vi "Read Acceleration.vi"(8 "error in (no error)":errorcluster, 11 "Sync 2-Axis Stage Controller in":refnum<class "Sync 2-Axis Stage Controller.lvclass">) -> (0 "error out":errorcluster, 1 "Y Acceleration":dbl, 2 "X Acceleration":dbl, 3 "Sync 2-Axis Stage Controller out":refnum<class "Sync 2-Axis Stage Controller.lvclass">)   [LabVIEW 2022 SP3, in "Sync 2-Axis Stage Controller.lvclass"]
uses:
  Sync 2-Axis Stage Controller.lvclass
  Sync 2-Axis Stage Controller.lvclass/Sync 2-Axis Stage Controller.ctl
  Axis Objects/iMotion Controller/iMotion Controller.lvclass
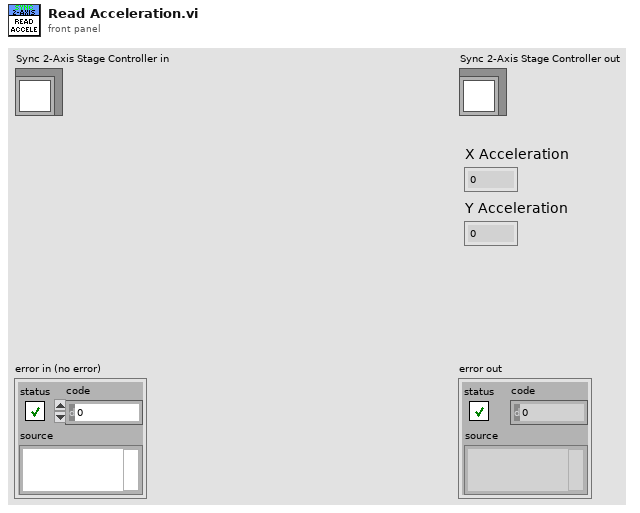
[diagram p1: front panel]
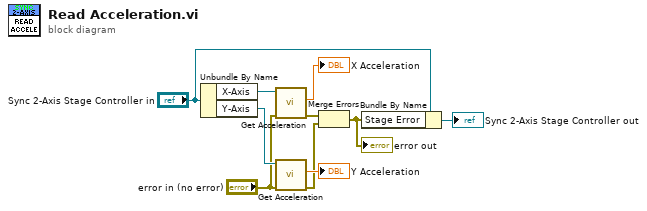
[diagram p0: block diagram]
diagram:
  n1 = Unbundle By Name("Sync 2-Axis Stage Controller in") -> ("X-Axis"=w9:refnum<class "iMotion Controller.lvclass">, "Y-Axis"=w8:refnum<class "iMotion Controller.lvclass">)
  n2 = call-dynamic "Get Acceleration.vi"("error in (no error)"="error in (no error)", "iMotion Controller in"=w9) -> ("error out"=w5:errorcluster, "Acceleration"=→"X Acceleration":dbl)  [unwired: 7 in, 1 out]
  n3 = call-dynamic "Get Acceleration.vi"("error in (no error)"="error in (no error)", "iMotion Controller in"=w8) -> ("error out"=w4:errorcluster, "Acceleration"=→"Y Acceleration":dbl)  [unwired: 7 in, 1 out]
  n4 = Merge Errors(w5, w4) -> (w1:errorcluster)
  "error out" <- w1
  n5 = Bundle By Name(cluster="Sync 2-Axis Stage Controller in", "Stage Error"=w1) -> (→"Sync 2-Axis Stage Controller out":refnum<class "Sync 2-Axis Stage Controller.lvclass">)
